vi "Set dBm Impedance.vi"(8 "error in (no error)":errorcluster, 10 "dBm Impedance (0: 50 ohms)":u32(ring) items=["50 ohms", "75 ohms", "90 ohms", "100 ohms", "135 ohms", "150 ohms", "300 ohms", "600 ohms", "900 ohms", "1000 ohms", "1200 ohms"], 11 "VISA resource name":refnum<visa-resource-name>) -> (0 "error out":errorcluster, 3 "VISA resource name out":refnum<visa-resource-name>)   [LabVIEW 2011, in "Fluke 5XXX Series Multicalibrators.lvlib"]
doc: "This VI sets the impedance used for dBm outputs (ac volts).\n\nNote:\n\nThis VI is available only for instrument model 5520A."
uses:
  Fluke 5XXX Series Multicalibrators.lvlib
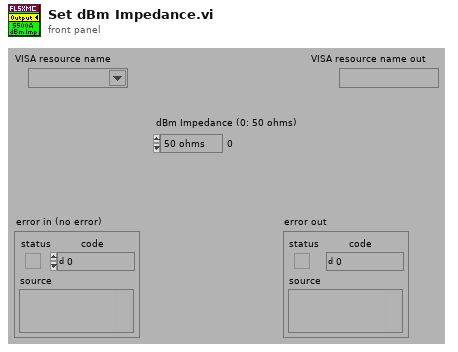
[diagram p1: front panel]
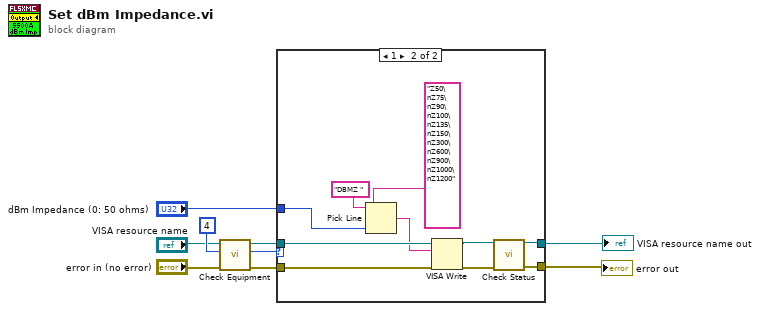
[diagram p0: block diagram]
diagram:
  n1 = call "Check Equipment.vi"("error in (no error)"="error in (no error)", "Bit Mask"=4 ("Numeric"), "VISA resource name"="VISA resource name") -> ("error out"=w8:errorcluster, "Present?"=w7:u32, "VISA resource name out"=w6:refnum<visa-resource-name>)  [unwired: 6 in]
  n2 = case shown="1" w7 {
    tunnel: "dBm Impedance (0: 50 ohms)" -> [_ w16]
    tunnel: [w10 w12] -> w2
    tunnel: w8 -> [w11 w19]
    tunnel: w6 -> [w10 w18]
    tunnel: [w11 w15] -> w1
    frame 0, Default {
    }
    frame 1 {
      n3 = Pick Line(string ("")="DBMZ " ("Reset Command"), multi-line string="Z50\nZ75\nZ90\nZ100\nZ135\nZ150\nZ300\nZ600\nZ900\nZ1000\nZ1200", line index=w16) -> (output string=w17:string)
      n4 = VISA Write(VISA resource name=w18, write buffer=w17, error in (no error)=w19) -> (VISA resource name out=w13:refnum<visa-resource-name>, error out=w14:errorcluster)  [unwired: 1 out]
      n5 = call "Check Status.vi"("VISA resource name"=w13, "error in (no error)"=w14) -> ("VISA resource name out"=w12:refnum<visa-resource-name>, "error out"=w15:errorcluster)  [unwired: 12 in]
    }
  }
  "VISA resource name out" <- w2
  "error out" <- w1
